vi "Validate Alias.vi"(10 "Alias":string) -> (2 "Valid Alias":bool)   [LabVIEW 2020]
uses:
  <vilib>/regexp/Match Regular Expression.xnode
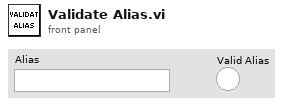
[diagram p1: front panel]
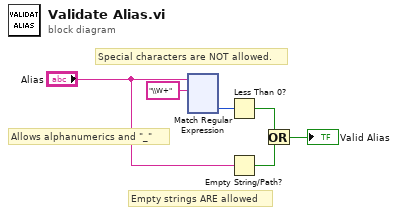
[diagram p0: block diagram]
diagram:
  # "Allows alphanumerics and \"_\""
  # "Empty strings ARE allowed"
  # "Special characters are NOT allowed."
  n1 = xnode "Match Regular Expression"("input string"="Alias", "regular expression"="\\W+") -> ("offset past match"=w4:i32)  [unwired: 4 in, 4 out]
  n2 = Less Than 0?(x=w4) -> (x < 0?=w3:bool)
  n3 = Empty String/Path?(string/path="Alias") -> (empty?=w2:bool)
  n4 = Or(x=w3, y=w2) -> (x .or. y?=→"Valid Alias":bool)
